vi "UpdateActualDepsList.vi"(6 "StatusIndicator Ref":refnum<vi>, 7 "LibraryNames":string[](array[string]), 8 "error in (no error)":errorcluster, 9 "ActualDependencies File Path":path=path "E:/sw-deps-monitor/Source/ActualDependencies/ActualDepsList.adeps", 10 "BuildSpecs Folder Path":path=path "E:/sw-deps-monitor/Source/BuildSpecs", 11 "Source Folder Path":path=path "E:/sw-deps-monitor/Source") -> (0 "error out":errorcluster)   [LabVIEW 2023, in "Reusables.lvlib"]
uses:
  Reusables/Reusables.lvlib
  <userlib>/_OpenG.lib/file/file.llb/openg_file.lvlib
  <vilib>/Utility/config.llb/NI_LVConfig.lvlib
panel:
  out "Status Indicator":string
  # "Leave Empty to update all Libraries"
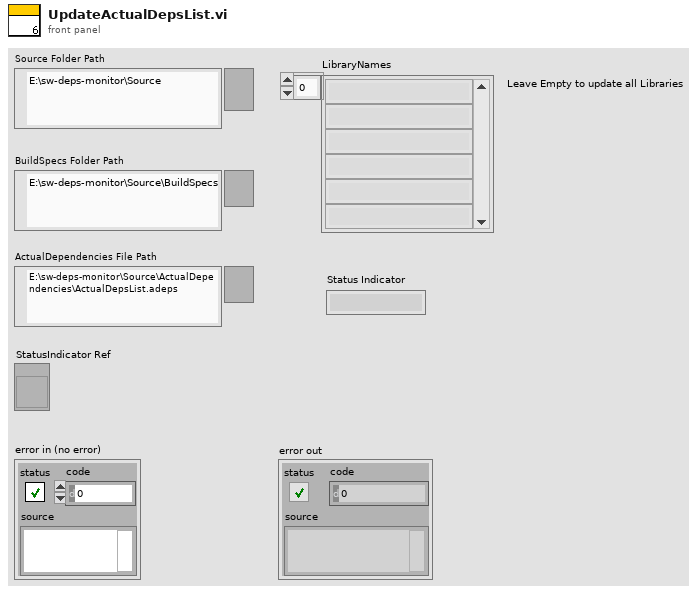
[diagram p1: front panel]
types:
  T1 = typedef "NI_LVConfig.lvlib/Config Data RefNum.ctl" = refnum<k1>
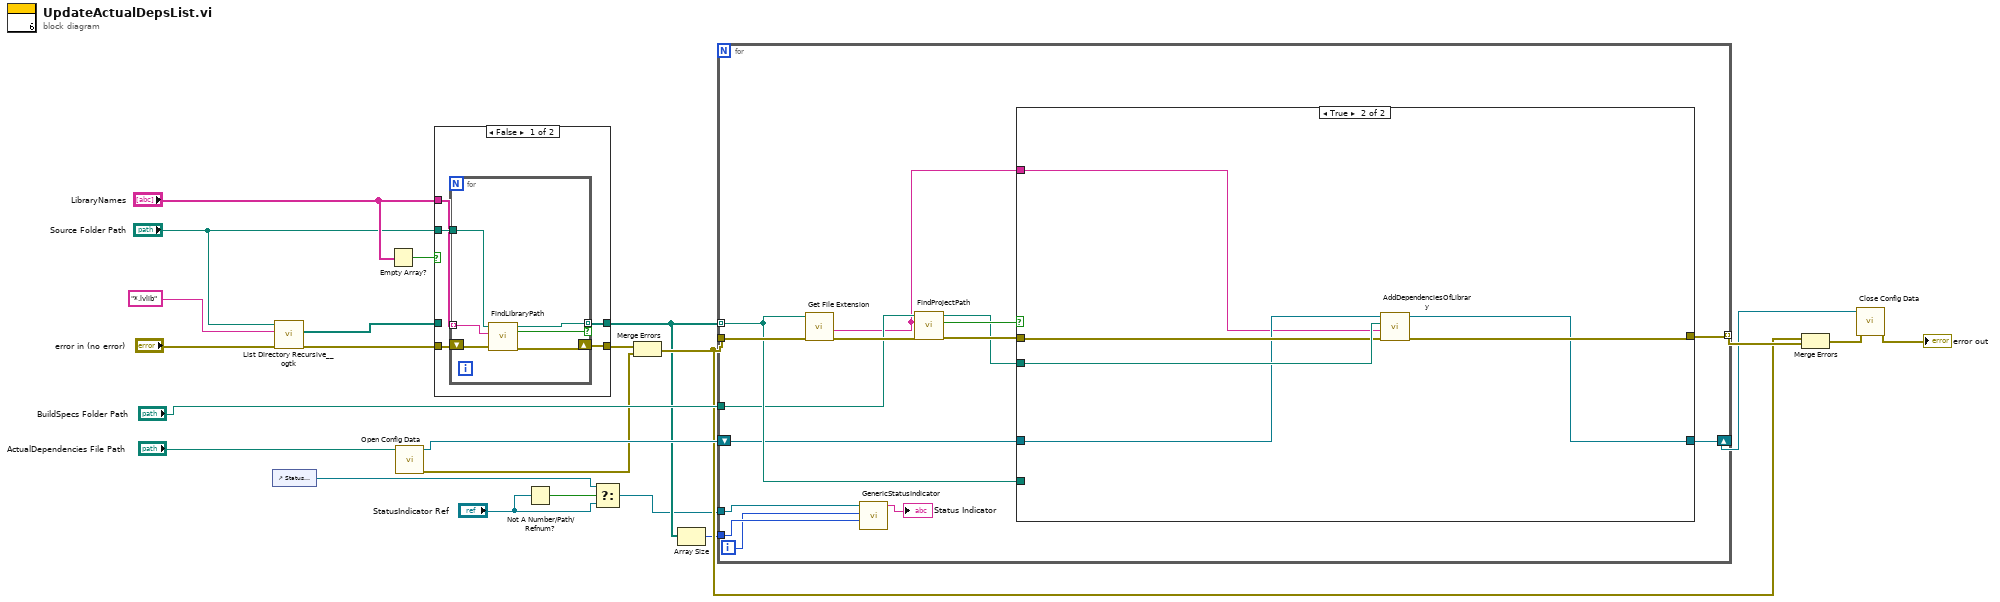
[diagram p0: block diagram]
diagram:
  n1 = control-ref of="Status Indicator"() -> (w3:refnum<vi>)
  n2 = call <userlib>:"List Directory Recursive__ogtk.vi"("error in (no error)"="error in (no error)", "pattern"="*.lvlib", "Path"="Source Folder Path") -> ("error out"=w12:errorcluster, "file paths"=w10:path[])  [unwired: 5 in, 2 out]
  n3 = Empty Array?(array="LibraryNames") -> (empty?=w11:bool)
  n4 = call <vilib>:"Open Config Data.vi"("configuration file path"="ActualDependencies File Path") -> ("error out"=w14:errorcluster, "refnum"=w18:T1)  [unwired: 8 in, 1 out]
  n5 = case shown="False" w11 {
    tunnel: w12 -> [w28 w35]
    tunnel: w10 -> [_ w36]
    tunnel: [w25 w36] -> w6
    tunnel: "LibraryNames" -> [w26 _]
    tunnel: "Source Folder Path" -> [w27 _]
    tunnel: [w24 w35] -> w7
    frame False {
      n6 = for {
        tunnel: w27 -> [w33]
        tunnel: w26 -> [w32] mode=indexing
        shift-right: [w31] -> w24
        shift-left: w28 -> [w34]
        tunnel: [w30] -> w25 mode=indexing if=w29
        n7 = call "FindLibraryPath.vi"("error in (no error)"=w34, "Library Name"=w32, "Source Folder Path"=w33) -> ("error out"=w31:errorcluster, "Found?"=w29:bool, "Library Path"=w30:path)  [unwired: 6 in]
      }
    }
    frame True {
    }
  }
  n8 = Not A Number/Path/Refnum?(number/path/refnum="StatusIndicator Ref") -> (NaN/Path/Refnum?=w4:bool)
  n9 = Select(t=w3, s=w4, f="StatusIndicator Ref") -> (s? t:f=w1:refnum<vi>)
  n10 = Merge Errors(w7, w14) -> (w13:errorcluster)
  n11 = Array Size(array=w6) -> (size(s)=w5:i32)
  n12 = for {
    tunnel: w13 -> [w51]
    tunnel: w6 -> [w49] mode=indexing
    tunnel: "BuildSpecs Folder Path" -> [w47]
    tunnel: [w50] -> w21 mode=indexing
    shift-right: [w42] -> w15
    shift-left: w18 -> [w43]
    tunnel: w1 -> [w40]
    tunnel: w5 -> [w39]
    i -> [w38]
    n13 = call <vilib>:"Get File Extension.vi"("error in (no error)"=w51, "file"=w49) -> ("error out"=w48:errorcluster, "filename without extension"=w41:string)  [unwired: 5 in, 3 out]
    n14 = call "GenericStatusIndicator.vi"("Total"=w39, "Current Iteration"=w38, "String in"=w40) -> ("Status"=→"Status Indicator":string)  [unwired: 8 in]
    n15 = call "FindProjectPath.vi"("error in (no error)"=w48, "Library Name"=w41, "Build Specs Folder Path"=w47) -> ("error out"=w45:errorcluster, "Found?"=w46:bool, "Project Path"=w44:path)  [unwired: 6 in]
    n16 = case shown="True" w46 {
      tunnel: w45 -> [w53 w58]
      tunnel: w49 -> [_ _]
      tunnel: [w53 w57] -> w50
      tunnel: w44 -> [_ w59]
      tunnel: w43 -> [w52 w56]
      tunnel: [w52 w55] -> w42
      tunnel: w41 -> [_ w54]
      frame False {
      }
      frame True {
        n17 = call "AddDependenciesOfLibrary.vi"("error in (no error)"=w58, "LibraryName"=w54, "Project Path"=w59, "Config Refnum in"=w56) -> ("error out"=w57:errorcluster, "Config Refnum out"=w55:T1)  [unwired: 6 in]
      }
    }
  }
  n18 = Merge Errors(w13, w21) -> (w17:errorcluster)
  n19 = call <vilib>:"Close Config Data.vi"("error in (no error)"=w17, "refnum"=w15) -> ("error out"=→"error out":errorcluster)  [unwired: 8 in, 1 out]
